vi "HardwareInit.vi"() -> ()   [LabVIEW 2026]
uses:
  01_Typen/GameCommandTypeDef.ctl
  <vilib>/MakerHub/LINX/Public/Peripherals/Digital/Digital Read 1 Chan.vi
  <vilib>/MakerHub/LINX/Public/Peripherals/Digital/Digital Read N Chans.vi
  <vilib>/MakerHub/LINX/Private/Local IO/LinxDigitalRead.vi
  <vilib>/MakerHub/LINX/Public/Utilities/Check Channel.vi
  <vilib>/MakerHub/LINX/Public/Utilities/Open Serial.vi
  <vilib>/MakerHub/LINX/Private/Utilties/Generate Error.vi
  <vilib>/MakerHub/LINX/LMH-LINX.lvlib
panel:
  out "Boolean 4":bool
  out "Boolean 3":bool
  out "Boolean 2":bool
  out "Boolean":bool
  in  "Input Pins":u8[](array[numeric])
  in  "Stop":bool
  in  "Serial Port":refnum<visa-resource-name>="N/A"
  # "Button 1"
  # "Button 2"
  # "Button 3"
  # "Button 4"
  # "Please use the Stop-Button to stop the VI. Otherwise the VI might break!"
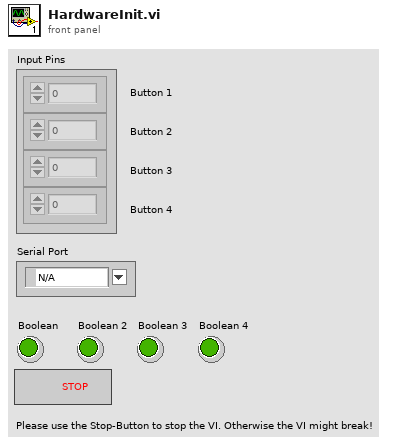
[diagram p1: front panel]
types:
  T1 = typedef "LMH-LINX.lvlib/LINX Ref.ctl" = cluster{"IO":T2, "Interface":T3, "LINX Device Config":T4}
  T2 = typedef "LMH-LINX.lvlib/Platform.ctl" = enum16{"Remote", "Local"}
  T3 = typedef "LMH-LINX.lvlib/Interface.ctl" = enum16{"Serial", "TCP"}
  T4 = typedef "LMH-LINX.lvlib/Device.lvlib/LINX Device Config.ctl" = cluster{"Interface":T3, "COM Port":refnum<visa-resource-name>, "TCP Configuration":T5, "Device Family":u8, "Device ID":u8, "Device Name":string, "TCP Ref":refnum<k5>, "Channels":T6}
  T5 = typedef "LMH-LINX.lvlib/Device.lvlib/TCP Config.ctl" = cluster{"IP Address":string, "Port":u16}
  T6 = typedef "LMH-LINX.lvlib/Channels.ctl" = cluster{"DI":u8[], "DO":u8[], "AI":u8[], "AO":u8[], "PWM":u8[], "QE":u8[], "UART":u8[], "I2C 2":u8[], "SPI":u8[], "CAN":u8[], "Servo":u8[], "AI Ref (V)":dbl, "AI Resolution (Bits)":u8, "AO Ref (V)":dbl, "AO Resolution (Bits)":u8}
  T7 = typedef "GameCommandTypeDef.ctl" = enum16{"NoCommand", "Rotate", "MoveLeft", "MoveRight"}
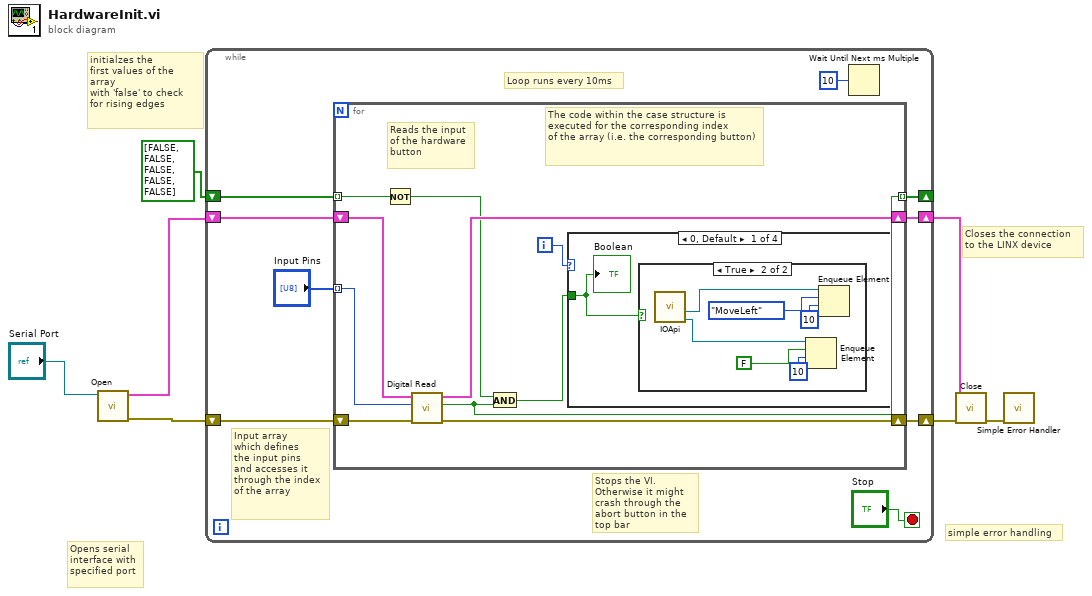
[diagram p0: block diagram]
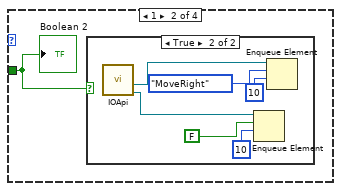
[diagram p3: hidden frame]
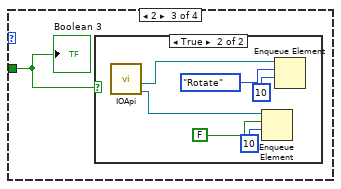
[diagram p5: hidden frame]
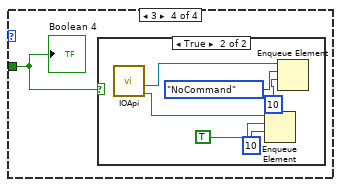
[diagram p7: hidden frame]
diagram:
  # "simple error handling"
  # "Closes the connection\nto the LINX device"
  # "initialzes the\nfirst values of the array\nwith 'false' to check\nfor rising edges"
  # "Opens serial\ninterface with\nspecified port"
  n1 = call-poly <vilib>:"Open.vi"("Serial Port"="Serial Port") -> ("Error Out"=w2:errorcluster, "LINX Resource"=w1:T1)  [unwired: 8 in, 1 out]
  n2 = while {
    shift-right: [w15] -> w5
    shift-left: w1 -> [w12]
    shift-right: [w13] -> w4
    shift-left: w2 -> [w14]
    shift-right: [w11] -> _
    shift-left: bool[] [FALSE, FALSE, FALSE, FALSE, FALSE] -> [w10]
    stop <- "Stop" stop-if-true
    # "Loop runs every 10ms"
    # "Input array\nwhich defines\nthe input pins\nand accesses it\nthrough the index\nof the array"
    # "Stops the VI.\nOtherwise it might crash through the abort button in the top bar"
    n3 = for {
      shift-right: [w22] -> w15
      shift-left: w12 -> [w25]
      shift-right: [w23] -> w13
      shift-left: w14 -> [w24]
      tunnel: [w20] -> w11 mode=indexing
      tunnel: w10 -> [w21] mode=indexing
      tunnel: "Input Pins" -> [w17] mode=indexing
      i -> [w26]
      # "The code within the case structure is\nexecuted for the corresponding index\nof the array (i.e. the corresponding button)"
      # "Reads the input\nof the hardware\nbutton"
      n4 = Not(x=w21) -> (.not. x?=w19:bool)
      n5 = call-poly <vilib>:"Digital Read.vi"("Error In"=w24, "DI Channel"=w17, "LINX Resource"=w25) -> ("Error Out"=w23:errorcluster, "DI Value"=w20:bool, "LINX Resource"=w22:T1)  [unwired: 6 in]
      n6 = And(x=w19, y=w20) -> (x .and. y?=w18:bool)
      n7 = case shown="0, Default" w26 {
        tunnel: w18 -> [w27 w34 w41 w48]
        frame 0, Default {
          n8 = case shown="True" w27 {
            frame False {
            }
            frame True {
              n9 = call "IOApi.vi"() -> ("Reset Queue Ref"=w31:refnum<queue>, "GameCommand out Queue Ref"=w33:refnum<queue>)  [unwired: 9 in, 1 out]
              n10 = Enqueue Element(queue=w31, element=FALSE ("Reset From Hardware"), timeout in ms (-1)=10) -> ()  [unwired: 1 in, 3 out]
              n11 = Enqueue Element(queue=w33, element=GameCommandTypeDef."MoveLeft" ("GameCommand From Hardware"), timeout in ms (-1)=10) -> ()  [unwired: 1 in, 3 out]
            }
          }
          "Boolean" <- w27
        }
        frame 1 {
          n12 = case shown="True" w34 {
            frame False {
            }
            frame True {
              n13 = call "IOApi.vi"() -> ("Reset Queue Ref"=w38:refnum<queue>, "GameCommand out Queue Ref"=w40:refnum<queue>)  [unwired: 9 in, 1 out]
              n14 = Enqueue Element(queue=w38, element=FALSE ("Reset From Hardware"), timeout in ms (-1)=10) -> ()  [unwired: 1 in, 3 out]
              n15 = Enqueue Element(queue=w40, element=GameCommandTypeDef."MoveRight" ("GameCommand From Hardware"), timeout in ms (-1)=10) -> ()  [unwired: 1 in, 3 out]
            }
          }
          "Boolean 2" <- w34
        }
        frame 2 {
          n16 = case shown="True" w41 {
            frame False {
            }
            frame True {
              n17 = call "IOApi.vi"() -> ("Reset Queue Ref"=w45:refnum<queue>, "GameCommand out Queue Ref"=w47:refnum<queue>)  [unwired: 9 in, 1 out]
              n18 = Enqueue Element(queue=w45, element=FALSE ("Reset From Hardware"), timeout in ms (-1)=10) -> ()  [unwired: 1 in, 3 out]
              n19 = Enqueue Element(queue=w47, element=GameCommandTypeDef."Rotate" ("GameCommand From Hardware"), timeout in ms (-1)=10) -> ()  [unwired: 1 in, 3 out]
            }
          }
          "Boolean 3" <- w41
        }
        frame 3 {
          n20 = case shown="True" w48 {
            frame False {
            }
            frame True {
              n21 = call "IOApi.vi"() -> ("Reset Queue Ref"=w52:refnum<queue>, "GameCommand out Queue Ref"=w54:refnum<queue>)  [unwired: 9 in, 1 out]
              n22 = Enqueue Element(queue=w52, element=TRUE ("Reset From Hardware"), timeout in ms (-1)=10) -> ()  [unwired: 1 in, 3 out]
              n23 = Enqueue Element(queue=w54, element=GameCommandTypeDef."NoCommand" ("GameCommand From Hardware"), timeout in ms (-1)=10) -> ()  [unwired: 1 in, 3 out]
            }
          }
          "Boolean 4" <- w48
        }
      }
    }
    n24 = Wait Until Next ms Multiple(millisecond multiple=u32 10 ("milliseconds to wait")) -> ()  [unwired: 1 out]
  }
  n25 = call <vilib>:"Close.vi"("Error In"=w4, "LINX Resource"=w5) -> ("Error Out"=w6:errorcluster)  [unwired: 9 in]
  n26 = call <vilib>:"Simple Error Handler.vi"("error in (no error)"=w6) -> ()  [unwired: 4 in, 5 out]
